vi "Do Core.vi"(8 "error in (no error)":errorcluster, 9 "Actor in":refnum<class "Actor.lvclass">, 11 "Reply Message":refnum<class "Remove View with Reply.lvclass">) -> (0 "error out":errorcluster, 1 "Actor out":refnum<class "Actor.lvclass">, 2 "Reply":variant)   [LabVIEW 2023, in "GUI Views.lvlib" / "Remove View with Reply.lvclass"]
doc: "(<B>Filename</B>: Actor Framework.lvlib:Reply Msg.lvclass:Do Core.vi)\n\nDefines what an actor does when it receives <B>Reply Message</B>. This method also defines the <B>Reply</B> that is returned to the actor that sent <B>Reply Message</B>.\n\nBy default, this method does nothing, and <B>Reply</B> is the ancestor Message class. A child class must override this method to define behavior and specify a child of the Message class to return in the <B>Reply</B> output."
uses:
  Remove View with Reply.lvclass
  <vilib>/ActorFramework/Actor/Actor.lvclass
  GUI Container/GUI Container.lvclass
  C:/Program Files/National Instruments/LabVIEW 2023/vi.lib/ActorFramework/Actor/Actor.lvclass
  Remove View with Reply.lvclass/Remove View with Reply.ctl
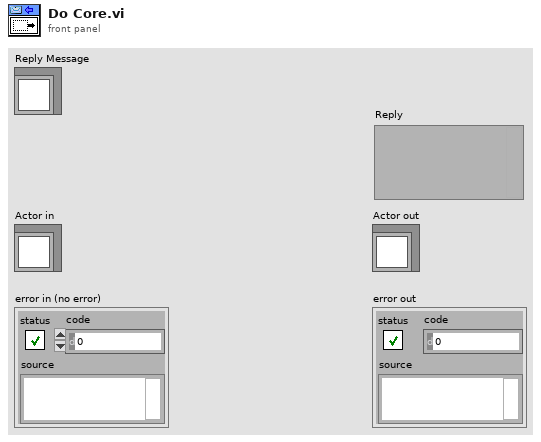
[diagram p1: front panel]
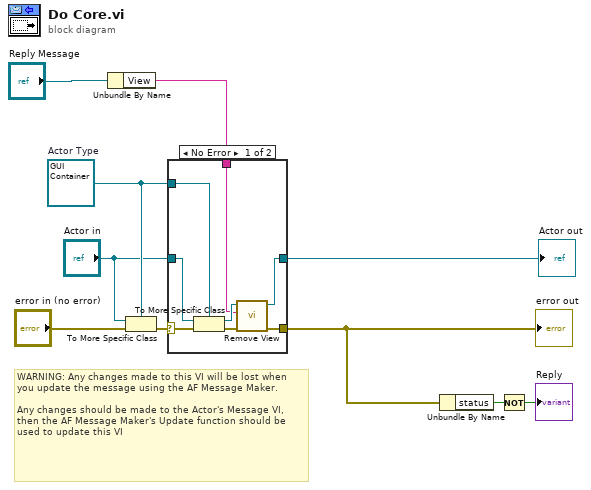
[diagram p0: block diagram]
diagram:
  w9 = refnum<class "GUI Container.lvclass"> refnum  # Actor Type
  # "WARNING: Any changes made to this VI will be lost when you update the message using the AF Message Maker.\n\nAny changes should be made to the Actor's Message VI, then the AF Message Maker's Update function should be used to update this VI"
  n1 = Unbundle By Name("Reply Message") -> ("View"=w1:string)
  n2 = To More Specific Class(target class=w9, reference="Actor in", error in="error in (no error)") -> (error out=w10:errorcluster)  [unwired: 1 out]
  n3 = case shown="No Error" w10 {
    selector: w10 -> [w18 w20]
    tunnel: [w13 w20] -> w5
    tunnel: [w12 w19] -> w7
    tunnel: "Actor in" -> [w17 w19]
    tunnel: w9 -> [w16 _]
    tunnel: w1 -> [w11 _]
    frame No Error {
      n4 = To More Specific Class ("Actor Cast")(target class=w16, reference=w17, error in=w18) -> (specific class reference=w15:refnum<class "GUI Container.lvclass">, error out=w14:errorcluster)
      n5 = call "Remove View.vi"("error in (no error)"=w14, "View"=w11, "GUI Container View Actor in"=w15) -> ("error out"=w13:errorcluster, "GUI Container View Actor out"=w12:refnum<class "GUI Container.lvclass">)  [unwired: 7 in]
    }
    frame Error {
    }
  }
  "error out" <- w5
  "Actor out" <- w7
  n6 = Unbundle By Name(w5) -> ("status"=w4:bool)
  n7 = Not(x=w4) -> (.not. x?=→"Reply":bool)
